vi "MaxEye_ATE_New_Load Configuration_Load to Variant.vi"(8 "error in (no error)":errorcluster, 10 "File Data":string, 11 "Variant In":variant) -> (0 "error out":errorcluster, 3 "Variant Out":variant)   [LabVIEW 2021]
uses:
  <vilib>/Utility/Data Type/NI_Data Type.lvlib
  <userlib>/_OpenG.lib/lvdata/lvdata.llb/openg_variant.lvlib
panel:
  out "Numeric":i32
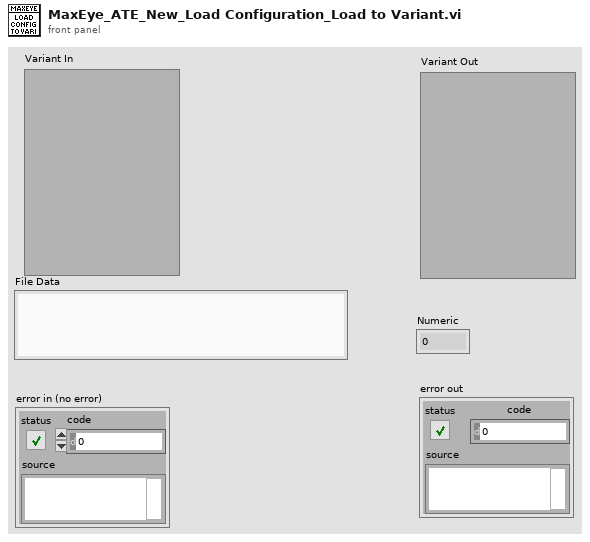
[diagram p1: front panel]
types:
  T1 = typedef "NI_Data Type.lvlib/Data Type.ctl" = enum8{"Invalid Type", "Void", "I8", "I16", "I32", "I64", "U8", "U16", "U32", "U64", "Single Float", "Double Float", "Extended Float", "Single Complex", "Double Complex", "Extended Complex", "Enum U8", "Enum U16", "Enum U32", "Enum U64", "Single Float With Unit", "Double Float With Unit", "Extended Float With Unit", "Single Complex with Unit", "Double Complex with Unit", "Extended Complex with Unit", "Boolean", "String", "Path", "Picture", "Tag", "Array", "Cluster", "Variant", "LV Variant", "Waveform", "Timestamp", "Digital Waveform", "Digital Data", "ExpressData", "Refnum", "External Data", "VI", "Poly VI", "LabVIEW Class Instance", "Fixed Point", "Set Collection", "Map Collection"}
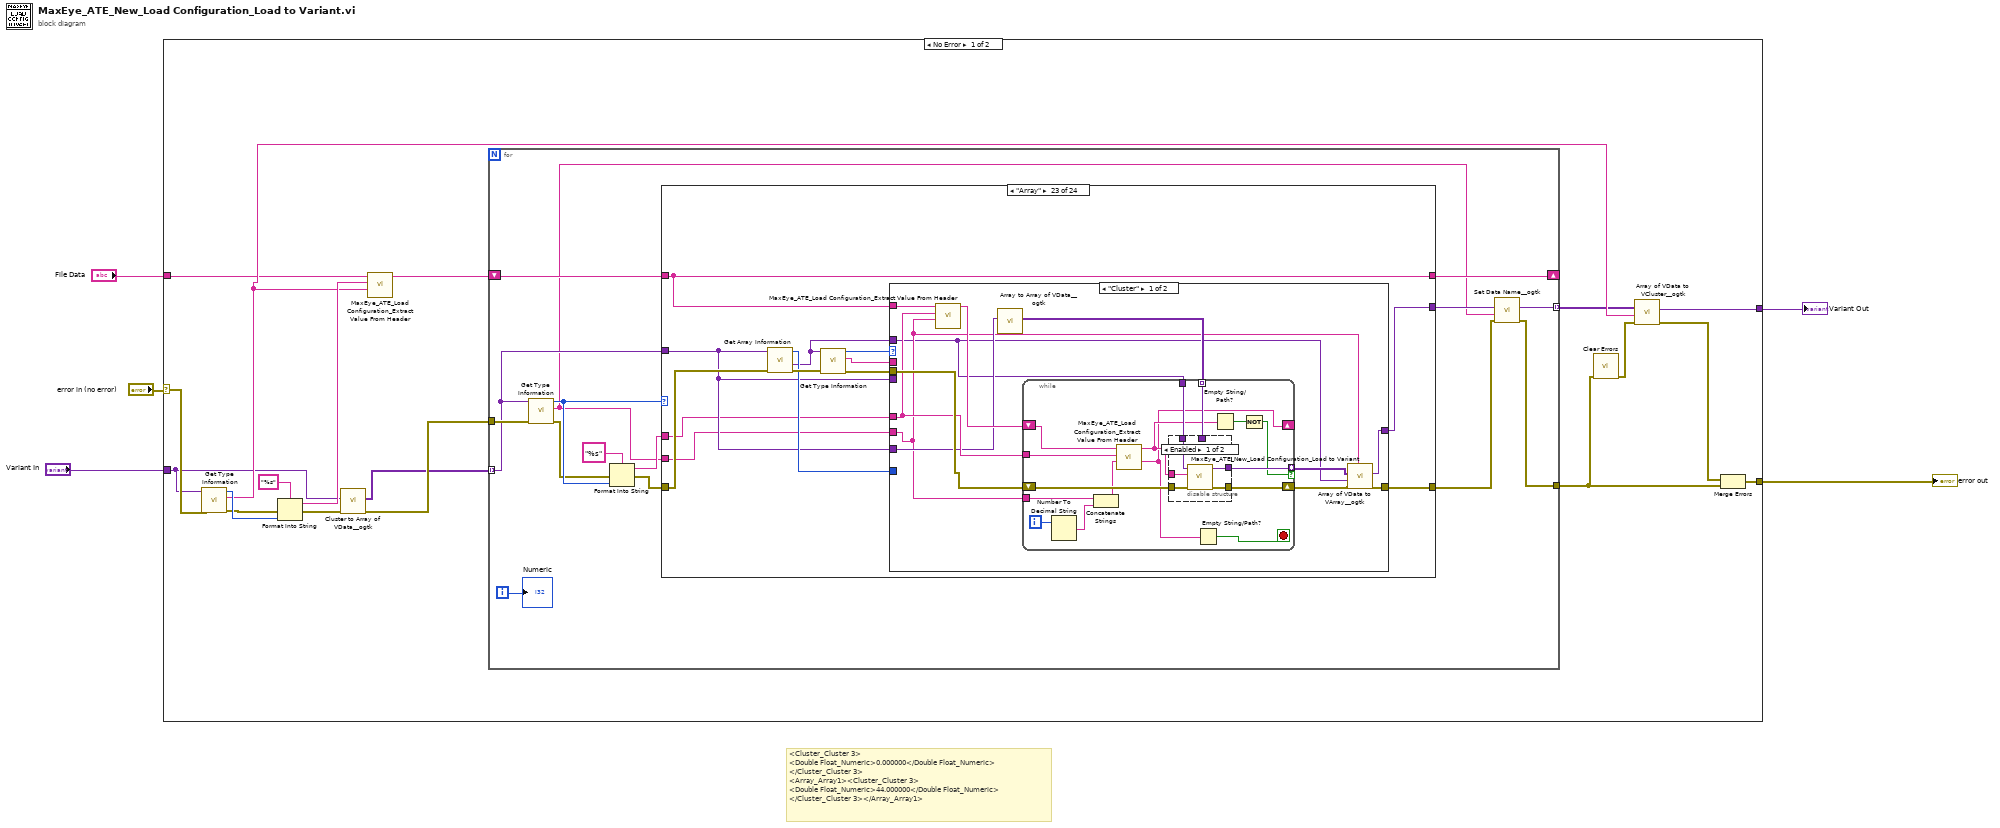
[diagram p0: block diagram]
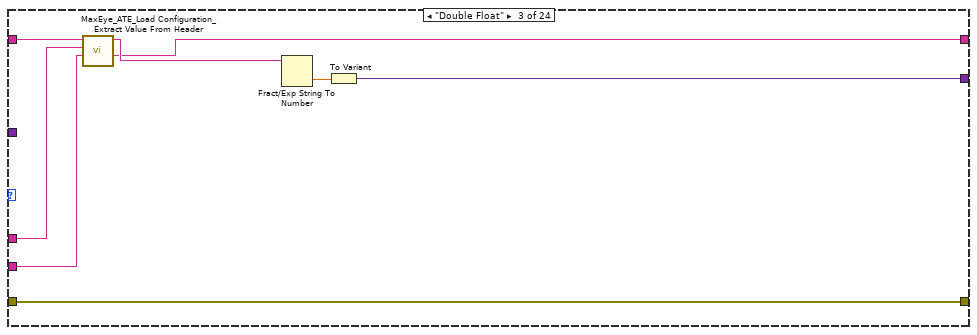
[diagram p4: hidden frame]
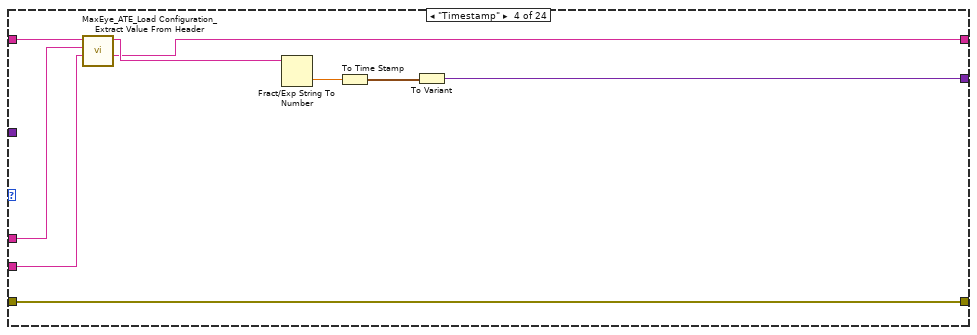
[diagram p5: hidden frame]
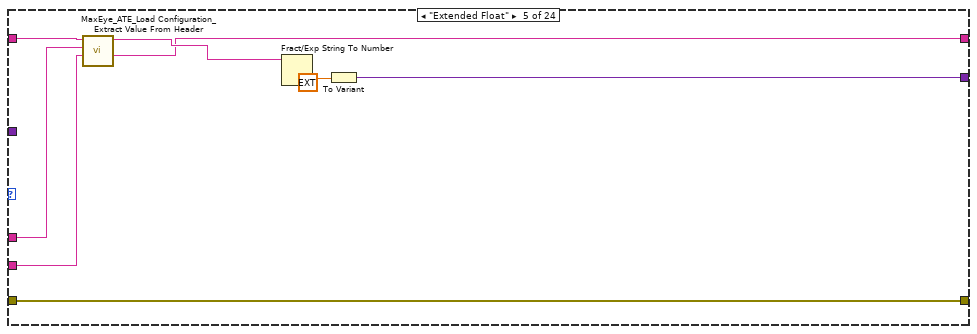
[diagram p6: hidden frame]
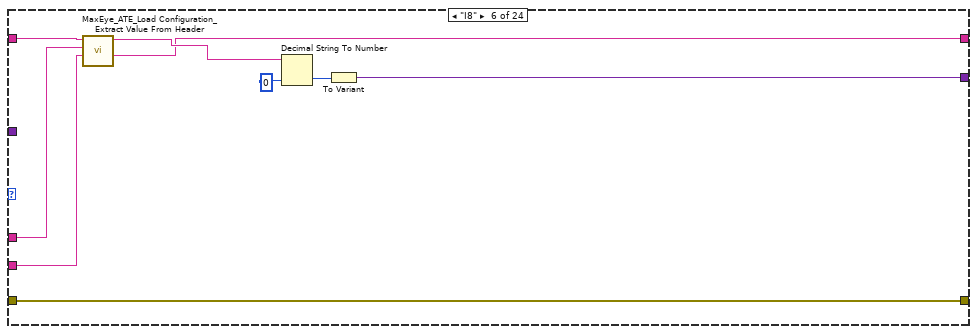
[diagram p7: hidden frame]
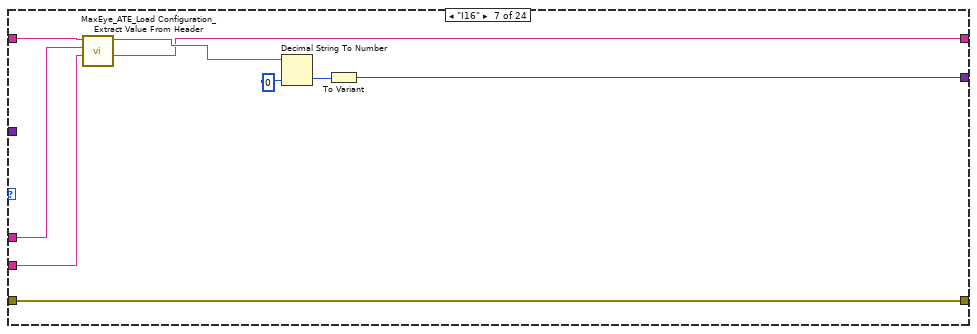
[diagram p8: hidden frame]
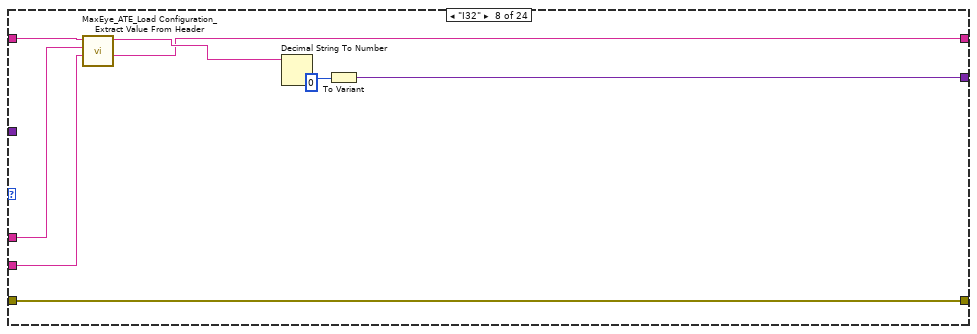
[diagram p9: hidden frame]
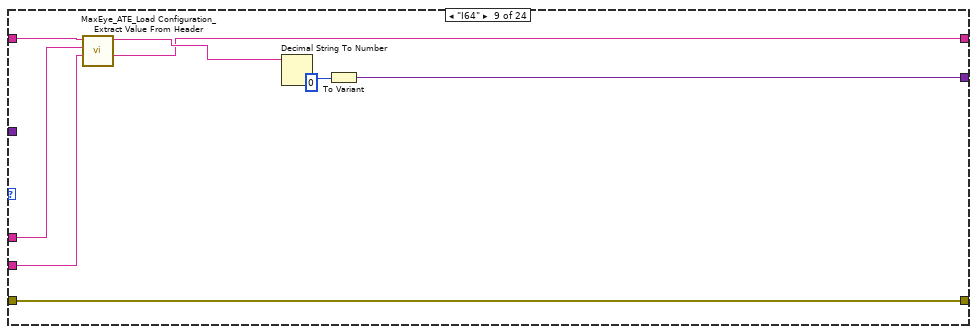
[diagram p10: hidden frame]
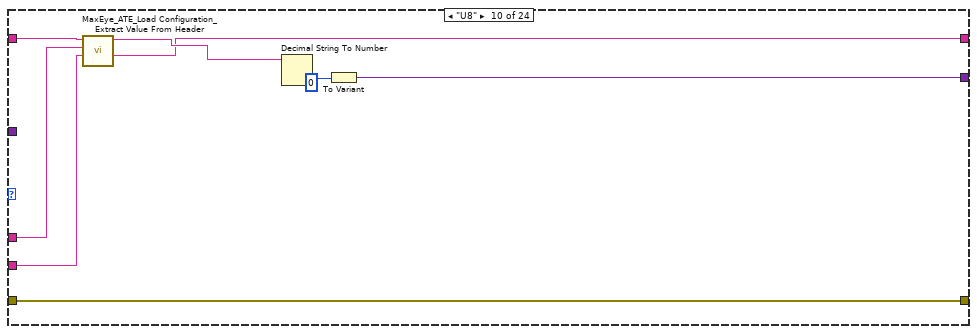
[diagram p11: hidden frame]
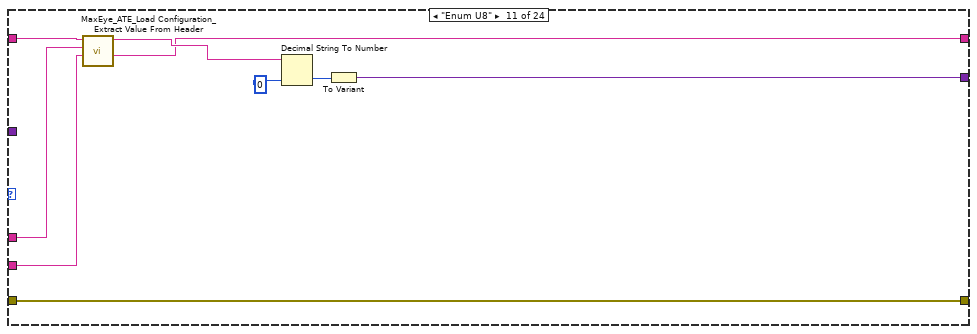
[diagram p12: hidden frame]
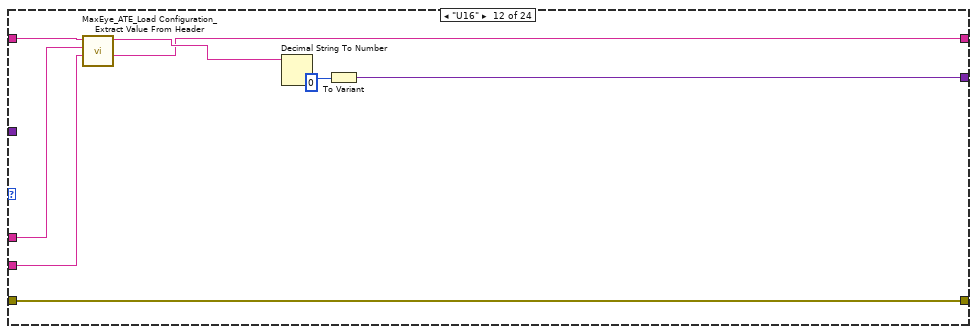
[diagram p13: hidden frame]
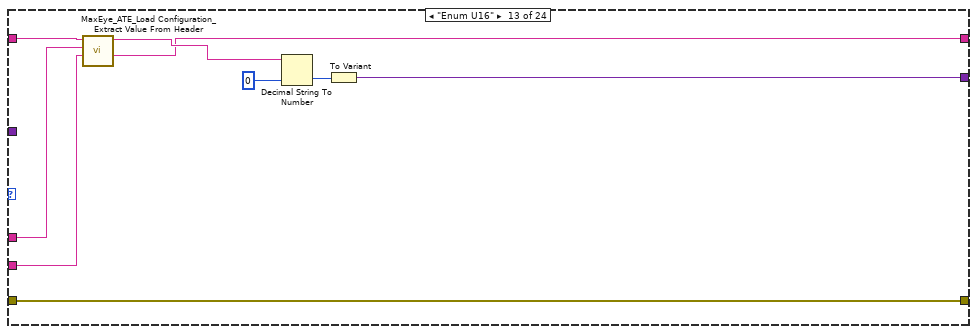
[diagram p14: hidden frame]
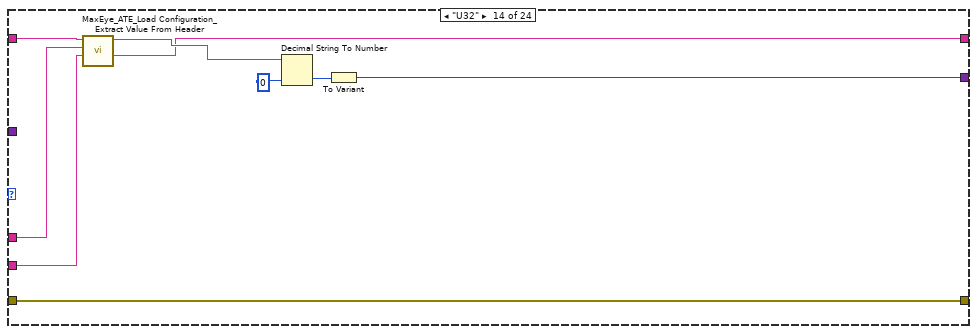
[diagram p15: hidden frame]
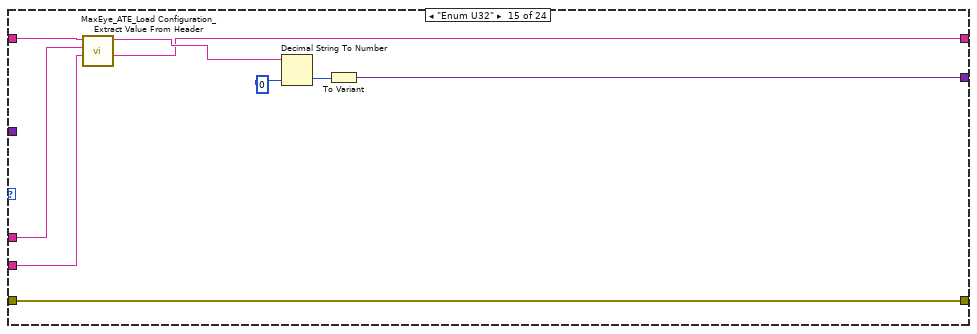
[diagram p16: hidden frame]
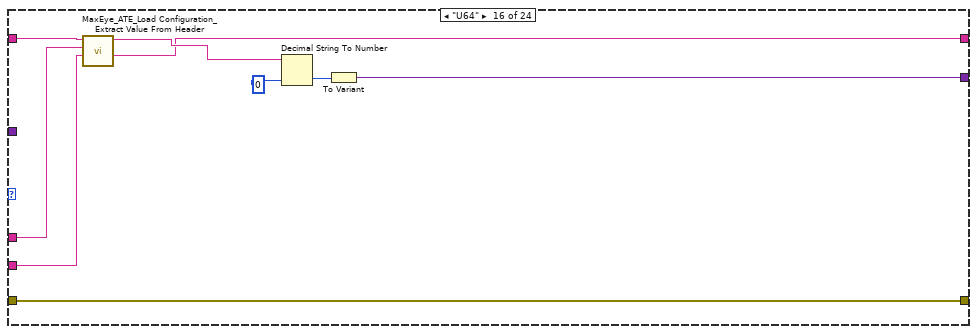
[diagram p17: hidden frame]
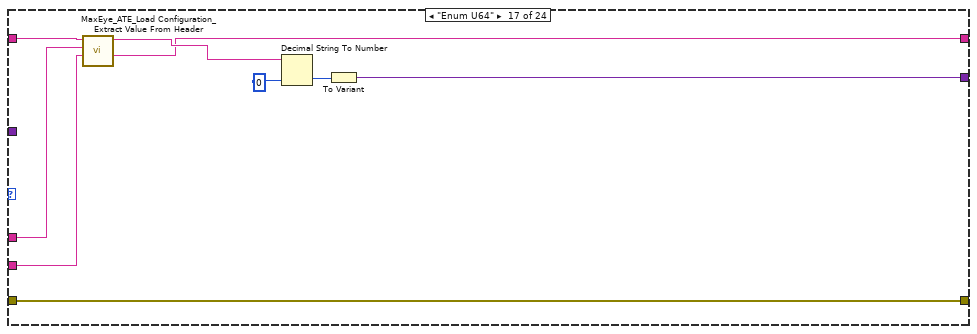
[diagram p18: hidden frame]
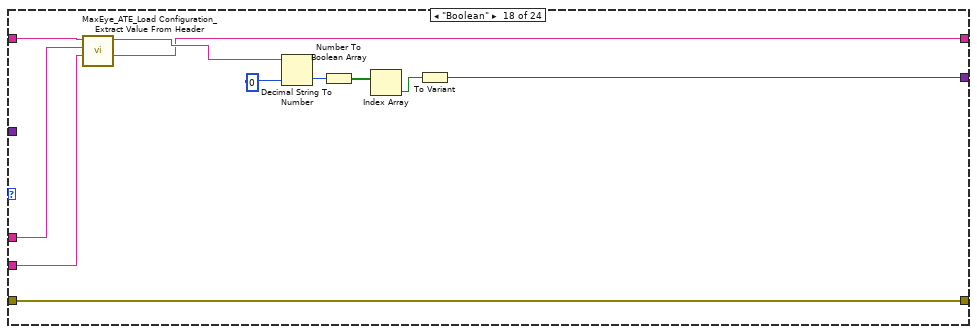
[diagram p19: hidden frame]
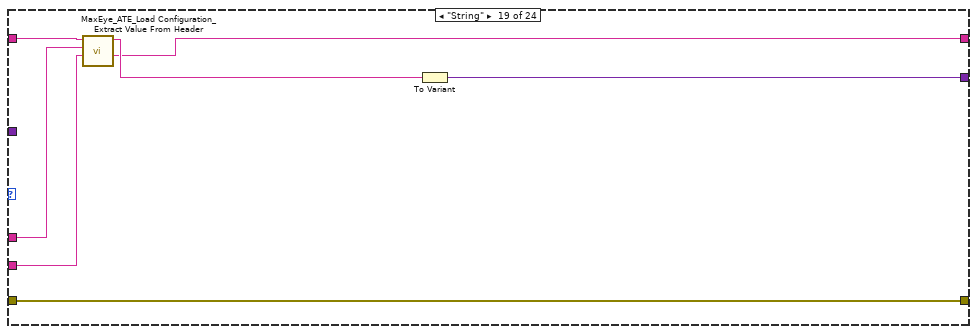
[diagram p20: hidden frame]
diagram:
  # "<Cluster_Cluster 3>\n<Double Float_Numeric>0.000000</Double Float_Numeric>\n</Cluster_Cluster 3>\n<Array_Array1><Cluster_Cluster 3>\n<Double Float_Numeric>44.000000</Double Float_Numeric>\n</Cluster_Cluster 3></Array_Array1>"
  n1 = case shown="No Error" "error in (no error)" {
    selector: "error in (no error)" -> [w23 w736]
    tunnel: "File Data" -> [w7 _]
    tunnel: [w12 w736] -> w4
    tunnel: "Variant In" -> [w8 _]
    tunnel: [w9 _] -> w3
    frame No Error {
      n2 = call <vilib>:"Get Type Information.vi"("error in (no error)"=w23, "variant"=w8) -> ("error out"=w20:errorcluster, "name"=w15:string, "type"=w22:T1)  [unwired: 5 in, 2 out]
      n3 = Format Into String(format string="%s", error in=w20, w22) -> (resulting string=w16:string, error out=w18:errorcluster)  [unwired: 1 in]
      n4 = call <userlib>:"Cluster to Array of VData__ogtk.vi"("error in (no error)"=w18, "Cluster"=w8) -> ("error out"=w19:errorcluster, "Array of VData"=w14:variant[])  [unwired: 8 in]
      n5 = call "MaxEye_ATE_Load Configuration_Extract Value From Header.vi"("Label Name"=w15, "Class Name"=w16, "File Data in"=w7) -> ("File Data out"=w6:string)  [unwired: 7 in, 1 out]
      n6 = for {
        tunnel: w19 -> [w38]
        shift-right: [w36] -> _
        shift-left: w6 -> [w37]
        tunnel: [w28] -> w11
        tunnel: w14 -> [w30] mode=indexing
        tunnel: [w29] -> w13 mode=indexing
        i -> [w24]
        n7 = call <vilib>:"Get Type Information.vi"("error in (no error)"=w38, "variant"=w30) -> ("error out"=w31:errorcluster, "name"=w26:string, "type"=w34:T1)  [unwired: 5 in, 2 out]
        n8 = Format Into String(format string="%s", error in=w31, w34) -> (resulting string=w33:string, error out=w32:errorcluster)  [unwired: 1 in]
        n9 = case shown="\"Array\"" w34 {
          tunnel: w32 -> [w39 w41 w50 w59 w68 w77 w86 w95 w104 w113 w122 w131 w140 w149 w158 w167 w176 w187 w194 w202 w209 w246 w265 w730]
          tunnel: w37 -> [w40 w42 w48 w57 w65 w74 w83 w92 w101 w110 w119 w128 w137 w146 w155 w164 w173 w184 w191 w199 w207 w244 w254 w723]
          tunnel: [w40 w42 w45 w54 w61 w70 w79 w88 w97 w106 w115 w124 w133 w142 w151 w160 w169 w180 w188 w196 w206 w243 w254 w724] -> w36
          tunnel: [w39 w41 w50 w59 w68 w77 w86 w95 w104 w113 w122 w131 w140 w149 w158 w167 w176 w187 w194 w202 w209 w246 w260 w729] -> w25
          tunnel: w26 -> [_ _ w43 w52 w66 w75 w84 w93 w102 w111 w120 w129 w138 w147 w156 w165 w174 w185 w192 w200 w203 w240 w258 w726]
          tunnel: w33 -> [_ _ w49 w58 w67 w76 w85 w94 w103 w112 w121 w130 w139 w148 w157 w166 w175 w186 w193 w201 w208 w245 w255 w727]
          tunnel: w30 -> [_ _ _ _ _ _ _ _ _ _ _ _ _ _ _ _ _ _ _ _ _ _ w259 w728]
          tunnel: [_ _ w44 w53 w62 w71 w80 w89 w98 w107 w116 w125 w134 w143 w152 w161 w170 w181 w189 w197 w205 w242 w256 w725] -> w27
          frame "Invalid Type", Default {
          }
          frame "Void" {
          }
          frame "Double Float" {
            n10 = call "MaxEye_ATE_Load Configuration_Extract Value From Header.vi"("Label Name"=w43, "Class Name"=w49, "File Data in"=w48) -> ("File Data Remaining"=w45:string, "File Data out"=w47:string)  [unwired: 7 in]
            n11 = Fract/Exp String To Number(string=w47) -> (number=w46:dbl)  [unwired: 3 in, 1 out]
            n12 = To Variant(anything=w46) -> (Variant=w44:variant)
          }
          frame "Timestamp" {
            n13 = call "MaxEye_ATE_Load Configuration_Extract Value From Header.vi"("Label Name"=w52, "Class Name"=w58, "File Data in"=w57) -> ("File Data Remaining"=w54:string, "File Data out"=w56:string)  [unwired: 7 in]
            n14 = Fract/Exp String To Number(string=w56) -> (number=w55:dbl)  [unwired: 3 in, 1 out]
            n15 = To Time Stamp(1:w55) -> (0:w51:timestamp)
            n16 = To Variant(anything=w51) -> (Variant=w53:variant)
          }
          frame "Extended Float" {
            n17 = call "MaxEye_ATE_Load Configuration_Extract Value From Header.vi"("Label Name"=w66, "Class Name"=w67, "File Data in"=w65) -> ("File Data Remaining"=w61:string, "File Data out"=w64:string)  [unwired: 7 in]
            n18 = Fract/Exp String To Number(string=w64, default (0 dbl)=ext 0.0 ("default (0 DBL)")) -> (number=w63:ext)  [unwired: 2 in, 1 out]
            n19 = To Variant(anything=w63) -> (Variant=w62:variant)
          }
          frame "I8" {
            n20 = call "MaxEye_ATE_Load Configuration_Extract Value From Header.vi"("Label Name"=w75, "Class Name"=w76, "File Data in"=w74) -> ("File Data Remaining"=w70:string, "File Data out"=w73:string)  [unwired: 7 in]
            n21 = Decimal String To Number(string=w73, default (0L)=i8 0 ("default (0 I32)")) -> (number=w72:i8)  [unwired: 1 in, 1 out]
            n22 = To Variant(anything=w72) -> (Variant=w71:variant)
          }
          frame "I16" {
            n23 = call "MaxEye_ATE_Load Configuration_Extract Value From Header.vi"("Label Name"=w84, "Class Name"=w85, "File Data in"=w83) -> ("File Data Remaining"=w79:string, "File Data out"=w82:string)  [unwired: 7 in]
            n24 = Decimal String To Number(string=w82, default (0L)=i16 0 ("default (0 I32)")) -> (number=w81:i16)  [unwired: 1 in, 1 out]
            n25 = To Variant(anything=w81) -> (Variant=w80:variant)
          }
          frame "I32" {
            n26 = call "MaxEye_ATE_Load Configuration_Extract Value From Header.vi"("Label Name"=w93, "Class Name"=w94, "File Data in"=w92) -> ("File Data Remaining"=w88:string, "File Data out"=w91:string)  [unwired: 7 in]
            n27 = Decimal String To Number(string=w91, default (0L)=0 ("default (0 I32)")) -> (number=w90:i32)  [unwired: 1 in, 1 out]
            n28 = To Variant(anything=w90) -> (Variant=w89:variant)
          }
          frame "I64" {
            n29 = call "MaxEye_ATE_Load Configuration_Extract Value From Header.vi"("Label Name"=w102, "Class Name"=w103, "File Data in"=w101) -> ("File Data Remaining"=w97:string, "File Data out"=w100:string)  [unwired: 7 in]
            n30 = Decimal String To Number(string=w100, default (0L)=i64 0 ("default (0 I32)")) -> (number=w99:i64)  [unwired: 1 in, 1 out]
            n31 = To Variant(anything=w99) -> (Variant=w98:variant)
          }
          frame "U8" {
            n32 = call "MaxEye_ATE_Load Configuration_Extract Value From Header.vi"("Label Name"=w111, "Class Name"=w112, "File Data in"=w110) -> ("File Data Remaining"=w106:string, "File Data out"=w109:string)  [unwired: 7 in]
            n33 = Decimal String To Number(string=w109, default (0L)=u8 0 ("default (0 I32)")) -> (number=w108:u8)  [unwired: 1 in, 1 out]
            n34 = To Variant(anything=w108) -> (Variant=w107:variant)
          }
          frame "Enum U8" {
            n35 = call "MaxEye_ATE_Load Configuration_Extract Value From Header.vi"("Label Name"=w120, "Class Name"=w121, "File Data in"=w119) -> ("File Data Remaining"=w115:string, "File Data out"=w118:string)  [unwired: 7 in]
            n36 = Decimal String To Number(string=w118, default (0L)=u8 0 ("default (0 I32)")) -> (number=w117:u8)  [unwired: 1 in, 1 out]
            n37 = To Variant(anything=w117) -> (Variant=w116:variant)
          }
          frame "U16" {
            n38 = call "MaxEye_ATE_Load Configuration_Extract Value From Header.vi"("Label Name"=w129, "Class Name"=w130, "File Data in"=w128) -> ("File Data Remaining"=w124:string, "File Data out"=w127:string)  [unwired: 7 in]
            n39 = Decimal String To Number(string=w127, default (0L)=u16 0 ("default (0 I32)")) -> (number=w126:u16)  [unwired: 1 in, 1 out]
            n40 = To Variant(anything=w126) -> (Variant=w125:variant)
          }
          frame "Enum U16" {
            n41 = call "MaxEye_ATE_Load Configuration_Extract Value From Header.vi"("Label Name"=w138, "Class Name"=w139, "File Data in"=w137) -> ("File Data Remaining"=w133:string, "File Data out"=w136:string)  [unwired: 7 in]
            n42 = Decimal String To Number(string=w136, default (0L)=u16 0 ("default (0 I32)")) -> (number=w135:u16)  [unwired: 1 in, 1 out]
            n43 = To Variant(anything=w135) -> (Variant=w134:variant)
          }
          frame "U32" {
            n44 = call "MaxEye_ATE_Load Configuration_Extract Value From Header.vi"("Label Name"=w147, "Class Name"=w148, "File Data in"=w146) -> ("File Data Remaining"=w142:string, "File Data out"=w145:string)  [unwired: 7 in]
            n45 = Decimal String To Number(string=w145, default (0L)=u32 0 ("default (0 I32)")) -> (number=w144:u32)  [unwired: 1 in, 1 out]
            n46 = To Variant(anything=w144) -> (Variant=w143:variant)
          }
          frame "Enum U32" {
            n47 = call "MaxEye_ATE_Load Configuration_Extract Value From Header.vi"("Label Name"=w156, "Class Name"=w157, "File Data in"=w155) -> ("File Data Remaining"=w151:string, "File Data out"=w154:string)  [unwired: 7 in]
            n48 = Decimal String To Number(string=w154, default (0L)=u32 0 ("default (0 I32)")) -> (number=w153:u32)  [unwired: 1 in, 1 out]
            n49 = To Variant(anything=w153) -> (Variant=w152:variant)
          }
          frame "U64" {
            n50 = call "MaxEye_ATE_Load Configuration_Extract Value From Header.vi"("Label Name"=w165, "Class Name"=w166, "File Data in"=w164) -> ("File Data Remaining"=w160:string, "File Data out"=w163:string)  [unwired: 7 in]
            n51 = Decimal String To Number(string=w163, default (0L)=u64 0 ("default (0 I32)")) -> (number=w162:u64)  [unwired: 1 in, 1 out]
            n52 = To Variant(anything=w162) -> (Variant=w161:variant)
          }
          frame "Enum U64" {
            n53 = call "MaxEye_ATE_Load Configuration_Extract Value From Header.vi"("Label Name"=w174, "Class Name"=w175, "File Data in"=w173) -> ("File Data Remaining"=w169:string, "File Data out"=w172:string)  [unwired: 7 in]
            n54 = Decimal String To Number(string=w172, default (0L)=u64 0 ("default (0 I32)")) -> (number=w171:u64)  [unwired: 1 in, 1 out]
            n55 = To Variant(anything=w171) -> (Variant=w170:variant)
          }
          frame "Boolean" {
            n56 = call "MaxEye_ATE_Load Configuration_Extract Value From Header.vi"("Label Name"=w185, "Class Name"=w186, "File Data in"=w184) -> ("File Data Remaining"=w180:string, "File Data out"=w183:string)  [unwired: 7 in]
            n57 = Decimal String To Number(string=w183, default (0L)=u64 0 ("default (0 I32)")) -> (number=w182:u64)  [unwired: 1 in, 1 out]
            n58 = Number To Boolean Array(number=w182) -> (Boolean array=w178:bool[])
            n59 = Index Array(array=w178) -> (element=w177:bool)  [unwired: 1 in]
            n60 = To Variant(anything=w177) -> (Variant=w181:variant)
          }
          frame "String" {
            n61 = call "MaxEye_ATE_Load Configuration_Extract Value From Header.vi"("Label Name"=w192, "Class Name"=w193, "File Data in"=w191) -> ("File Data Remaining"=w188:string, "File Data out"=w190:string)  [unwired: 7 in]
            n62 = To Variant(anything=w190) -> (Variant=w189:variant)
          }
          frame "Path" {
            n63 = call "MaxEye_ATE_Load Configuration_Extract Value From Header.vi"("Label Name"=w200, "Class Name"=w201, "File Data in"=w199) -> ("File Data Remaining"=w196:string, "File Data out"=w198:string)  [unwired: 7 in]
            n64 = String To Path(string=w198) -> (path=w195:path)
            n65 = To Variant(anything=w195) -> (Variant=w197:variant)
          }
          frame "Refnum" {
            n66 = call "MaxEye_ATE_Load Configuration_Extract Value From Header.vi"("Label Name"=w203, "Class Name"=w208, "File Data in"=w207) -> ("File Data Remaining"=w206:string, "File Data out"=w204:string)  [unwired: 7 in]
            n67 = case shown="\"USRP Device ID\"" w203 {
              tunnel: [w211 w214 w218 w222 w226 w230 w234 w238] -> w205
              tunnel: w204 -> [w210 w213 w217 w221 w225 w229 w233 w237]
              frame Default {
                n68 = To Variant(anything=w210) -> (Variant=w211:variant)
              }
              frame "VISA resource name" {
                w212 = refnum<visa-resource-name> refnum  # VISA resource name
                n69 = Type Cast(type=w212, x=w213) -> (*(type *) &x=w215:refnum<visa-resource-name>)
                n70 = To Variant(anything=w215) -> (Variant=w214:variant)
              }
              frame "USRP Device ID" {
                w216 = refnum<k15> refnum  # USRP Device ID
                n71 = Type Cast(type=w216, x=w217) -> (*(type *) &x=w219:refnum<k15>)
                n72 = To Variant(anything=w219) -> (Variant=w218:variant)
              }
              frame "XNET Interface" {
                w220 = refnum<k21> refnum  # XNET Interface
                n73 = Type Cast(type=w220, x=w221) -> (*(type *) &x=w223:refnum<k21>)
                n74 = To Variant(anything=w223) -> (Variant=w222:variant)
              }
              frame "XNET Database" {
                w224 = refnum<k21> refnum  # XNET Database
                n75 = Type Cast(type=w224, x=w225) -> (*(type *) &x=w227:refnum<k21>)
                n76 = To Variant(anything=w227) -> (Variant=w226:variant)
              }
              frame "XNET Frame" {
                w228 = refnum<k21> refnum  # XNET Frame
                n77 = Type Cast(type=w228, x=w229) -> (*(type *) &x=w231:refnum<k21>)
                n78 = To Variant(anything=w231) -> (Variant=w230:variant)
              }
              frame "XNET Signal" {
                w232 = refnum<k21> refnum  # XNET Signal
                n79 = Type Cast(type=w232, x=w233) -> (*(type *) &x=w235:refnum<k21>)
                n80 = To Variant(anything=w235) -> (Variant=w234:variant)
              }
              frame "XNET Session" {
                w236 = refnum<k21> refnum  # XNET Session
                n81 = Type Cast(type=w236, x=w237) -> (*(type *) &x=w239:refnum<k21>)
                n82 = To Variant(anything=w239) -> (Variant=w238:variant)
              }
            }
          }
          frame "Tag" {
            n83 = call "MaxEye_ATE_Load Configuration_Extract Value From Header.vi"("Label Name"=w240, "Class Name"=w245, "File Data in"=w244) -> ("File Data Remaining"=w243:string, "File Data out"=w241:string)  [unwired: 7 in]
            n84 = case shown="\"RIO Resource\"" w240 {
              tunnel: [w248 w251] -> w242
              tunnel: w241 -> [w247 w250]
              frame Default {
                n85 = To Variant(anything=w247) -> (Variant=w248:variant)
              }
              frame "RIO Resource" {
                w249 = tag ""  # RIO Resource
                n86 = Type Cast(type=w249, x=w250) -> (*(type *) &x=w252:tag)
                n87 = To Variant(anything=w252) -> (Variant=w251:variant)
              }
            }
          }
          frame "Array" {
            n88 = call <vilib>:"Get Array Information.vi"("error in (no error)"=w265, "variant"=w259) -> ("error out"=w264:errorcluster, "array element data type"=w257:variant, "number of dimensions"=w263:i32)  [unwired: 6 in, 1 out]
            n89 = call <vilib>:"Get Type Information.vi"("error in (no error)"=w264, "variant"=w257) -> ("error out"=w261:errorcluster, "name"=w253:string, "type"=w262:T1)  [unwired: 5 in, 2 out]
            n90 = case shown="\"Cluster\"" w262 {
              selector: w262 -> [_ w307]
              tunnel: w263 -> [_ w308]
              tunnel: w261 -> [w275 w303]
              tunnel: w255 -> [w274 w306]
              tunnel: w258 -> [w267 w305]
              tunnel: w259 -> [w271 w304]
              tunnel: [w273 w302] -> w260
              tunnel: w259 -> [_ _]
              tunnel: w254 -> [w277 w301]
              tunnel: [w272 w300] -> w256
              tunnel: w257 -> [w266 _]
              tunnel: w253 -> [_ _]
              frame "Cluster" {
                n91 = call "MaxEye_ATE_Load Configuration_Extract Value From Header.vi"("Label Name"=w267, "Class Name"=w274, "File Data in"=w277) -> ("File Data out"=w276:string)  [unwired: 7 in, 1 out]
                n92 = call <userlib>:"Array to Array of VData__ogtk.vi"("MultiD Array"=w271) -> ("1D Array of Variants"=w270:variant[])  [unwired: 9 in, 1 out]
                n93 = while {
                  shift-right: [w292] -> w269
                  shift-left: w275 -> [w293]
                  tunnel: w267 -> [w291]
                  tunnel: [w288] -> w268 mode=indexing if=w279
                  tunnel: w274 -> [w286]
                  tunnel: w266 -> [w284]
                  tunnel: w270 -> [w283] mode=indexing
                  shift-right: [w278] -> _
                  shift-left: w276 -> [w285]
                  i -> [w289]
                  stop <- w282 stop-if-true
                  n94 = Number To Decimal String(number=w289) -> (decimal integer string=w290:string)  [unwired: 1 in]
                  n95 = Concatenate Strings(w291, w290) -> (w287:string)
                  n96 = call "MaxEye_ATE_Load Configuration_Extract Value From Header.vi"("Label Name"=w287, "Class Name"=w286, "File Data in"=w285) -> ("File Data Remaining"=w278:string, "File Data out"=w281:string)  [unwired: 7 in]
                  n97 = disable-structure shown="Enabled" {
                    disable-tunnel: w293 -> [w298 _]
                    disable-tunnel: [w297 _] -> w292
                    disable-tunnel: [w296 w299] -> w288
                    disable-tunnel: w281 -> [w295 _]
                    disable-tunnel: w284 -> [w294 _]
                    disable-tunnel: w283 -> [_ w299]
                    frame Enabled {
                      n98 = call "MaxEye_ATE_New_Load Configuration_Load to Variant.vi"("error in (no error)"=w298, "File Data"=w295, "Variant In"=w294) -> ("error out"=w297:errorcluster, "Variant Out"=w296:variant)  [unwired: 7 in]
                    }
                    frame Disabled {
                    }
                  }
                  n99 = Empty String/Path?(string/path=w278) -> (empty?=w282:bool)
                  n100 = Empty String/Path?(string/path=w281) -> (empty?=w280:bool)
                  n101 = Not(x=w280) -> (.not. x?=w279:bool)
                }
                n102 = call <userlib>:"Array of VData to VArray__ogtk.vi"("Array Name"=w267, "error in (no error)"=w269, "Element Type (when empty)"=w266, "1D Array of VData"=w268) -> ("error out"=w273:errorcluster, "VArray"=w272:variant)  [unwired: 6 in]
              }
              frame "Void", Default {
                n103 = case shown="2" w308 {
                  tunnel: w307 -> [_ w317 w468 w599]
                  tunnel: w306 -> [_ w314 w465 w596]
                  tunnel: w305 -> [_ w313 w464 w595]
                  tunnel: w304 -> [_ _ _ _]
                  tunnel: w303 -> [w309 w316 w467 w598]
                  tunnel: [w309 w315 w466 w597] -> w302
                  tunnel: w301 -> [_ w312 w463 w594]
                  tunnel: [_ w310 w461 w592] -> w300
                  frame 0, Default {
                  }
                  frame 1 {
                    n104 = call "MaxEye_ATE_Load Configuration_Extract Value From Header.vi"("Label Name"=w313, "Class Name"=w314, "File Data in"=w312) -> ("File Data out"=w311:string)  [unwired: 7 in, 1 out]
                    n105 = case shown="\"String\"" w317 {
                      tunnel: w316 -> [w318 w325 w332 w339 w346 w353 w360 w367 w374 w381 w388 w395 w402 w409 w416 w423 w433 w441 w455 w460]
                      tunnel: [w318 w325 w332 w339 w346 w353 w360 w367 w374 w381 w388 w395 w402 w409 w416 w423 w433 w441 w455 w460] -> w315
                      tunnel: w311 -> [w324 w331 w338 w345 w352 w359 w366 w373 w380 w387 w394 w401 w408 w415 w422 w429 w438 w446 w459 _]
                      tunnel: [w319 w326 w333 w340 w347 w354 w361 w368 w375 w382 w389 w396 w403 w410 w417 w424 w434 w442 w456 _] -> w310
                      frame "I8" {
                        n106 = Spreadsheet String To Array(delimiter (Tab)=",", format string="%s", spreadsheet string=w324, array type (2D Dbl)=i8[] []) -> (array=w320:i8[])
                        n107 = To Variant(anything=w320) -> (Variant=w319:variant)
                      }
                      frame "I16" {
                        n108 = Spreadsheet String To Array(delimiter (Tab)=",", format string="%s", spreadsheet string=w331, array type (2D Dbl)=i16[] []) -> (array=w327:i16[])
                        n109 = To Variant(anything=w327) -> (Variant=w326:variant)
                      }
                      frame "I32" {
                        n110 = Spreadsheet String To Array(delimiter (Tab)=",", format string="%s", spreadsheet string=w338, array type (2D Dbl)=i32[] []) -> (array=w334:i32[])
                        n111 = To Variant(anything=w334) -> (Variant=w333:variant)
                      }
                      frame "I64" {
                        n112 = Spreadsheet String To Array(delimiter (Tab)=",", format string="%s", spreadsheet string=w345, array type (2D Dbl)=i64[] []) -> (array=w341:i64[])
                        n113 = To Variant(anything=w341) -> (Variant=w340:variant)
                      }
                      frame "U8" {
                        n114 = Spreadsheet String To Array(delimiter (Tab)=",", format string="%s", spreadsheet string=w352, array type (2D Dbl)=u8[] []) -> (array=w348:u8[])
                        n115 = To Variant(anything=w348) -> (Variant=w347:variant)
                      }
                      frame "Enum U8" {
                        n116 = Spreadsheet String To Array(delimiter (Tab)=",", format string="%s", spreadsheet string=w359, array type (2D Dbl)=u8[] []) -> (array=w355:u8[])
                        n117 = To Variant(anything=w355) -> (Variant=w354:variant)
                      }
                      frame "U16" {
                        n118 = Spreadsheet String To Array(delimiter (Tab)=",", format string="%s", spreadsheet string=w366, array type (2D Dbl)=u16[] []) -> (array=w362:u16[])
                        n119 = To Variant(anything=w362) -> (Variant=w361:variant)
                      }
                      frame "Enum U16" {
                        n120 = Spreadsheet String To Array(delimiter (Tab)=",", format string="%s", spreadsheet string=w373, array type (2D Dbl)=u16[] []) -> (array=w369:u16[])
                        n121 = To Variant(anything=w369) -> (Variant=w368:variant)
                      }
                      frame "U32" {
                        n122 = Spreadsheet String To Array(delimiter (Tab)=",", format string="%s", spreadsheet string=w380, array type (2D Dbl)=u32[] []) -> (array=w376:u32[])
                        n123 = To Variant(anything=w376) -> (Variant=w375:variant)
                      }
                      frame "Enum U32" {
                        n124 = Spreadsheet String To Array(delimiter (Tab)=",", format string="%s", spreadsheet string=w387, array type (2D Dbl)=u32[] []) -> (array=w383:u32[])
                        n125 = To Variant(anything=w383) -> (Variant=w382:variant)
                      }
                      frame "U64" {
                        n126 = Spreadsheet String To Array(delimiter (Tab)=",", format string="%s", spreadsheet string=w394, array type (2D Dbl)=u64[] []) -> (array=w390:u64[])
                        n127 = To Variant(anything=w390) -> (Variant=w389:variant)
                      }
                      frame "Enum U64" {
                        n128 = Spreadsheet String To Array(delimiter (Tab)=",", format string="%s", spreadsheet string=w401, array type (2D Dbl)=u64[] []) -> (array=w397:u64[])
                        n129 = To Variant(anything=w397) -> (Variant=w396:variant)
                      }
                      frame "Single Float" {
                        n130 = Spreadsheet String To Array(delimiter (Tab)=",", format string="%s", spreadsheet string=w408, array type (2D Dbl)=sgl[] []) -> (array=w404:sgl[])
                        n131 = To Variant(anything=w404) -> (Variant=w403:variant)
                      }
                      frame "Double Float" {
                        n132 = Spreadsheet String To Array(delimiter (Tab)=",", format string="%s", spreadsheet string=w415, array type (2D Dbl)=dbl[] []) -> (array=w411:dbl[])
                        n133 = To Variant(anything=w411) -> (Variant=w410:variant)
                      }
                      frame "Extended Float" {
                        n134 = Spreadsheet String To Array(delimiter (Tab)=",", format string="%s", spreadsheet string=w422, array type (2D Dbl)=ext[] []) -> (array=w418:ext[])
                        n135 = To Variant(anything=w418) -> (Variant=w417:variant)
                      }
                      frame "String" {
                        n136 = Spreadsheet String To Array(delimiter (Tab)=",", format string="%s", spreadsheet string=w429, array type (2D Dbl)=string[] []) -> (array=w425:string[])
                        n137 = To Variant(anything=w425) -> (Variant=w424:variant)
                      }
                      frame "Timestamp" {
                        n138 = Spreadsheet String To Array(delimiter (Tab)=",", format string="%s", spreadsheet string=w438, array type (2D Dbl)=string[] []) -> (array=w431:string[])
                        n139 = Fract/Exp String To Number(string=w431) -> (number=w432:dbl[])  [unwired: 3 in, 1 out]
                        n140 = To Time Stamp(1:w432) -> (0:w430:timestamp[])
                        n141 = To Variant(anything=w430) -> (Variant=w434:variant)
                      }
                      frame "Refnum" {
                        n142 = Spreadsheet String To Array(delimiter (Tab)=",", format string="%s", spreadsheet string=w446, array type (2D Dbl)=string[] []) -> (array=w439:string[])
                        n143 = for {
                          tunnel: [w448] -> w440 mode=indexing
                          tunnel: w439 -> [w447] mode=indexing
                          w449 = refnum<k21> refnum  # XNET Signal
                          n144 = Type Cast(type=w449, x=w447) -> (*(type *) &x=w448:refnum<k21>)
                        }
                        n145 = To Variant(anything=w440) -> (Variant=w442:variant)
                      }
                      frame "Boolean" {
                        n146 = Boolean To (0,1)(Boolean=bool[] []) -> (0, 1=w453:i16[])
                        n147 = Spreadsheet String To Array(delimiter (Tab)=",", format string="%s", spreadsheet string=w459, array type (2D Dbl)=w453) -> (array=w452:i16[])
                        n148 = Equal?(x=i16 1, y=w452) -> (x = y?=w450:bool[])
                        n149 = To Variant(anything=w450) -> (Variant=w456:variant)
                      }
                      frame "Void", Default {
                      }
                    }
                  }
                  frame 2 {
                    n150 = call "MaxEye_ATE_Load Configuration_Extract Value From Header.vi"("Label Name"=w464, "Class Name"=w465, "File Data in"=w463) -> ("File Data out"=w462:string)  [unwired: 7 in, 1 out]
                    n151 = case shown="\"String\"" w468 {
                      tunnel: w467 -> [w469 w476 w483 w490 w497 w504 w511 w518 w525 w532 w539 w546 w553 w560 w567 w574 w586 w591]
                      tunnel: [w469 w476 w483 w490 w497 w504 w511 w518 w525 w532 w539 w546 w553 w560 w567 w574 w586 w591] -> w466
                      tunnel: w462 -> [w475 w482 w489 w496 w503 w510 w517 w524 w531 w538 w545 w552 w559 w566 w573 w580 w590 _]
                      tunnel: [w470 w477 w484 w491 w498 w505 w512 w519 w526 w533 w540 w547 w554 w561 w568 w575 w587 _] -> w461
                      frame "I8" {
                        n152 = Spreadsheet String To Array(delimiter (Tab)=",", format string="%s", spreadsheet string=w475, array type (2D Dbl)=i8[][] []) -> (array=w471:i8[][])
                        n153 = To Variant(anything=w471) -> (Variant=w470:variant)
                      }
                      frame "I16" {
                        n154 = Spreadsheet String To Array(delimiter (Tab)=",", format string="%s", spreadsheet string=w482, array type (2D Dbl)=i16[][] []) -> (array=w478:i16[][])
                        n155 = To Variant(anything=w478) -> (Variant=w477:variant)
                      }
                      frame "I32" {
                        n156 = Spreadsheet String To Array(delimiter (Tab)=",", format string="%s", spreadsheet string=w489, array type (2D Dbl)=i32[][] []) -> (array=w485:i32[][])
                        n157 = To Variant(anything=w485) -> (Variant=w484:variant)
                      }
                      frame "I64" {
                        n158 = Spreadsheet String To Array(delimiter (Tab)=",", format string="%s", spreadsheet string=w496, array type (2D Dbl)=i64[][] []) -> (array=w492:i64[][])
                        n159 = To Variant(anything=w492) -> (Variant=w491:variant)
                      }
                      frame "U8" {
                        n160 = Spreadsheet String To Array(delimiter (Tab)=",", format string="%s", spreadsheet string=w503, array type (2D Dbl)=u8[][] []) -> (array=w499:u8[][])
                        n161 = To Variant(anything=w499) -> (Variant=w498:variant)
                      }
                      frame "Enum U8" {
                        n162 = Spreadsheet String To Array(delimiter (Tab)=",", format string="%s", spreadsheet string=w510, array type (2D Dbl)=u8[][] []) -> (array=w506:u8[][])
                        n163 = To Variant(anything=w506) -> (Variant=w505:variant)
                      }
                      frame "U16" {
                        n164 = Spreadsheet String To Array(delimiter (Tab)=",", format string="%s", spreadsheet string=w517, array type (2D Dbl)=u16[][] []) -> (array=w513:u16[][])
                        n165 = To Variant(anything=w513) -> (Variant=w512:variant)
                      }
                      frame "Enum U16" {
                        n166 = Spreadsheet String To Array(delimiter (Tab)=",", format string="%s", spreadsheet string=w524, array type (2D Dbl)=u16[][] []) -> (array=w520:u16[][])
                        n167 = To Variant(anything=w520) -> (Variant=w519:variant)
                      }
                      frame "U32" {
                        n168 = Spreadsheet String To Array(delimiter (Tab)=",", format string="%s", spreadsheet string=w531, array type (2D Dbl)=u32[][] []) -> (array=w527:u32[][])
                        n169 = To Variant(anything=w527) -> (Variant=w526:variant)
                      }
                      frame "Enum U32" {
                        n170 = Spreadsheet String To Array(delimiter (Tab)=",", format string="%s", spreadsheet string=w538, array type (2D Dbl)=u32[][] []) -> (array=w534:u32[][])
                        n171 = To Variant(anything=w534) -> (Variant=w533:variant)
                      }
                      frame "U64" {
                        n172 = Spreadsheet String To Array(delimiter (Tab)=",", format string="%s", spreadsheet string=w545, array type (2D Dbl)=u64[][] []) -> (array=w541:u64[][])
                        n173 = To Variant(anything=w541) -> (Variant=w540:variant)
                      }
                      frame "Enum U64" {
                        n174 = Spreadsheet String To Array(delimiter (Tab)=",", format string="%s", spreadsheet string=w552, array type (2D Dbl)=u64[][] []) -> (array=w548:u64[][])
                        n175 = To Variant(anything=w548) -> (Variant=w547:variant)
                      }
                      frame "Single Float" {
                        n176 = Spreadsheet String To Array(delimiter (Tab)=",", format string="%s", spreadsheet string=w559, array type (2D Dbl)=sgl[][] []) -> (array=w555:sgl[][])
                        n177 = To Variant(anything=w555) -> (Variant=w554:variant)
                      }
                      frame "Double Float" {
                        n178 = Spreadsheet String To Array(delimiter (Tab)=",", format string="%s", spreadsheet string=w566, array type (2D Dbl)=dbl[][] []) -> (array=w562:dbl[][])
                        n179 = To Variant(anything=w562) -> (Variant=w561:variant)
                      }
                      frame "Extended Float" {
                        n180 = Spreadsheet String To Array(delimiter (Tab)=",", format string="%s", spreadsheet string=w573, array type (2D Dbl)=ext[][] []) -> (array=w569:ext[][])
                        n181 = To Variant(anything=w569) -> (Variant=w568:variant)
                      }
                      frame "String" {
                        n182 = Spreadsheet String To Array(delimiter (Tab)=",", format string="%s", spreadsheet string=w580, array type (2D Dbl)=string[][] []) -> (array=w576:string[][])
                        n183 = To Variant(anything=w576) -> (Variant=w575:variant)
                      }
                      frame "Boolean" {
                        n184 = Boolean To (0,1)(Boolean=bool[][] []) -> (0, 1=w584:i16[][])
                        n185 = Spreadsheet String To Array(delimiter (Tab)=",", format string="%s", spreadsheet string=w590, array type (2D Dbl)=w584) -> (array=w583:i16[][])
                        n186 = Equal?(x=i16 1, y=w583) -> (x = y?=w581:bool[][])
                        n187 = To Variant(anything=w581) -> (Variant=w587:variant)
                      }
                      frame "Void", Default {
                      }
                    }
                  }
                  frame 3 {
                    n188 = call "MaxEye_ATE_Load Configuration_Extract Value From Header.vi"("Label Name"=w595, "Class Name"=w596, "File Data in"=w594) -> ("File Data out"=w593:string)  [unwired: 7 in, 1 out]
                    n189 = case shown="\"Double Float\"" w599 {
                      tunnel: w598 -> [w600 w607 w614 w621 w628 w635 w642 w649 w656 w663 w670 w677 w684 w691 w698 w705 w717 w722]
                      tunnel: [w600 w607 w614 w621 w628 w635 w642 w649 w656 w663 w670 w677 w684 w691 w698 w705 w717 w722] -> w597
                      tunnel: w593 -> [w606 w613 w620 w627 w634 w641 w648 w655 w662 w669 w676 w683 w690 w697 w704 w711 w721 _]
                      tunnel: [w601 w608 w615 w622 w629 w636 w643 w650 w657 w664 w671 w678 w685 w692 w699 w706 w718 _] -> w592
                      frame "I8" {
                        n190 = Spreadsheet String To Array(delimiter (Tab)=",", format string="%s", spreadsheet string=w606, array type (2D Dbl)=i8[][][] []) -> (array=w602:i8[][][])
                        n191 = To Variant(anything=w602) -> (Variant=w601:variant)
                      }
                      frame "I16" {
                        n192 = Spreadsheet String To Array(delimiter (Tab)=",", format string="%s", spreadsheet string=w613, array type (2D Dbl)=i16[][][] []) -> (array=w609:i16[][][])
                        n193 = To Variant(anything=w609) -> (Variant=w608:variant)
                      }
                      frame "I32" {
                        n194 = Spreadsheet String To Array(delimiter (Tab)=",", format string="%s", spreadsheet string=w620, array type (2D Dbl)=i32[][][] []) -> (array=w616:i32[][][])
                        n195 = To Variant(anything=w616) -> (Variant=w615:variant)
                      }
                      frame "I64" {
                        n196 = Spreadsheet String To Array(delimiter (Tab)=",", format string="%s", spreadsheet string=w627, array type (2D Dbl)=i64[][][] []) -> (array=w623:i64[][][])
                        n197 = To Variant(anything=w623) -> (Variant=w622:variant)
                      }
                      frame "U8" {
                        n198 = Spreadsheet String To Array(delimiter (Tab)=",", format string="%s", spreadsheet string=w634, array type (2D Dbl)=u8[][][] []) -> (array=w630:u8[][][])
                        n199 = To Variant(anything=w630) -> (Variant=w629:variant)
                      }
                      frame "Enum U8" {
                        n200 = Spreadsheet String To Array(delimiter (Tab)=",", format string="%s", spreadsheet string=w641, array type (2D Dbl)=u8[][][] []) -> (array=w637:u8[][][])
                        n201 = To Variant(anything=w637) -> (Variant=w636:variant)
                      }
                      frame "U16" {
                        n202 = Spreadsheet String To Array(delimiter (Tab)=",", format string="%s", spreadsheet string=w648, array type (2D Dbl)=u16[][][] []) -> (array=w644:u16[][][])
                        n203 = To Variant(anything=w644) -> (Variant=w643:variant)
                      }
                      frame "Enum U16" {
                        n204 = Spreadsheet String To Array(delimiter (Tab)=",", format string="%s", spreadsheet string=w655, array type (2D Dbl)=u16[][][] []) -> (array=w651:u16[][][])
                        n205 = To Variant(anything=w651) -> (Variant=w650:variant)
                      }
                      frame "U32" {
                        n206 = Spreadsheet String To Array(delimiter (Tab)=",", format string="%s", spreadsheet string=w662, array type (2D Dbl)=u32[][][] []) -> (array=w658:u32[][][])
                        n207 = To Variant(anything=w658) -> (Variant=w657:variant)
                      }
                      frame "Enum U32" {
                        n208 = Spreadsheet String To Array(delimiter (Tab)=",", format string="%s", spreadsheet string=w669, array type (2D Dbl)=u32[][][] []) -> (array=w665:u32[][][])
                        n209 = To Variant(anything=w665) -> (Variant=w664:variant)
                      }
                      frame "U64" {
                        n210 = Spreadsheet String To Array(delimiter (Tab)=",", format string="%s", spreadsheet string=w676, array type (2D Dbl)=u64[][][] []) -> (array=w672:u64[][][])
                        n211 = To Variant(anything=w672) -> (Variant=w671:variant)
                      }
                      frame "Enum U64" {
                        n212 = Spreadsheet String To Array(delimiter (Tab)=",", format string="%s", spreadsheet string=w683, array type (2D Dbl)=u64[][][] []) -> (array=w679:u64[][][])
                        n213 = To Variant(anything=w679) -> (Variant=w678:variant)
                      }
                      frame "Single Float" {
                        n214 = Spreadsheet String To Array(delimiter (Tab)=",", format string="%s", spreadsheet string=w690, array type (2D Dbl)=sgl[][][] []) -> (array=w686:sgl[][][])
                        n215 = To Variant(anything=w686) -> (Variant=w685:variant)
                      }
                      frame "Double Float" {
                        n216 = Spreadsheet String To Array(delimiter (Tab)=",", format string="%s", spreadsheet string=w697, array type (2D Dbl)=dbl[][][] []) -> (array=w693:dbl[][][])
                        n217 = To Variant(anything=w693) -> (Variant=w692:variant)
                      }
                      frame "Extended Float" {
                        n218 = Spreadsheet String To Array(delimiter (Tab)=",", format string="%s", spreadsheet string=w704, array type (2D Dbl)=ext[][][] []) -> (array=w700:ext[][][])
                        n219 = To Variant(anything=w700) -> (Variant=w699:variant)
                      }
                      frame "String" {
                        n220 = Spreadsheet String To Array(delimiter (Tab)=",", format string="%s", spreadsheet string=w711, array type (2D Dbl)=string[][][] []) -> (array=w707:string[][][])
                        n221 = To Variant(anything=w707) -> (Variant=w706:variant)
                      }
                      frame "Boolean" {
                        n222 = Boolean To (0,1)(Boolean=bool[][][] []) -> (0, 1=w715:i16[][][])
                        n223 = Spreadsheet String To Array(delimiter (Tab)=",", format string="%s", spreadsheet string=w721, array type (2D Dbl)=w715) -> (array=w714:i16[][][])
                        n224 = Equal?(x=i16 1, y=w714) -> (x = y?=w712:bool[][][])
                        n225 = To Variant(anything=w712) -> (Variant=w718:variant)
                      }
                      frame "Void", Default {
                      }
                    }
                  }
                }
              }
            }
          }
          frame "Cluster" {
            n226 = call "MaxEye_ATE_Load Configuration_Extract Value From Header.vi"("Label Name"=w726, "Class Name"=w727, "File Data in"=w723) -> ("File Data Remaining"=w724:string)  [unwired: 7 in, 1 out]
            n227 = disable-structure shown="Enabled" {
              disable-tunnel: w730 -> [w735 _]
              disable-tunnel: [w734 _] -> w729
              disable-tunnel: w728 -> [w733 _]
              disable-tunnel: w723 -> [w732 _]
              disable-tunnel: [w731 _] -> w725
              frame Enabled {
                n228 = call "MaxEye_ATE_New_Load Configuration_Load to Variant.vi"("error in (no error)"=w735, "File Data"=w732, "Variant In"=w733) -> ("error out"=w734:errorcluster, "Variant Out"=w731:variant)  [unwired: 7 in]
              }
              frame Disabled {
              }
            }
          }
        }
        n229 = call <userlib>:"Set Data Name__ogtk.vi"("error in (no error)"=w25, "Data Name"=w26, "Data"=w27) -> ("error out"=w28:errorcluster, "Renamed Data"=w29:variant)  [unwired: 7 in]
        "Numeric" <- w24
      }
      n230 = call <vilib>:"Clear Errors.vi"("error in (no error)"=w11) -> ("error out"=w10:errorcluster)  [unwired: 5 in, 1 out]
      n231 = call <userlib>:"Array of VData to VCluster__ogtk.vi"("error in (no error)"=w10, "Cluster Name"=w15, "Array"=w13) -> ("error out"=w17:errorcluster, "VCluster"=w9:variant)  [unwired: 7 in]
      n232 = Merge Errors(w17, w11) -> (w12:errorcluster)
    }
    frame Error {
    }
  }
  "error out" <- w4
  "Variant Out" <- w3
